vi "test_interpol.vi"() -> ()   [LabVIEW 2018]
uses:
  <vilib>/ptbypt/NI_PtbyPt.lvlib
panel:
  in  "sample length":i32=100
  in  "milliseconds to wait":u32
  in  "stop":bool
  out "Waveform Chart":dbl(graph)
  in  "x value":dbl format="%0.2f"
  in  "y":dbl format="%0.2f"
  out "Waveform Graph":dbl[](graph)
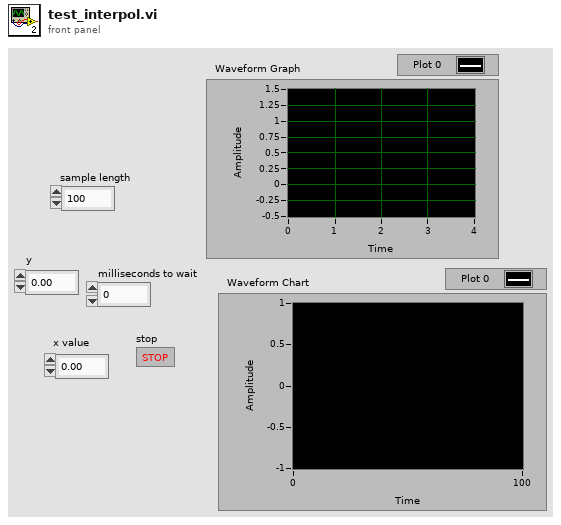
[diagram p1: front panel]
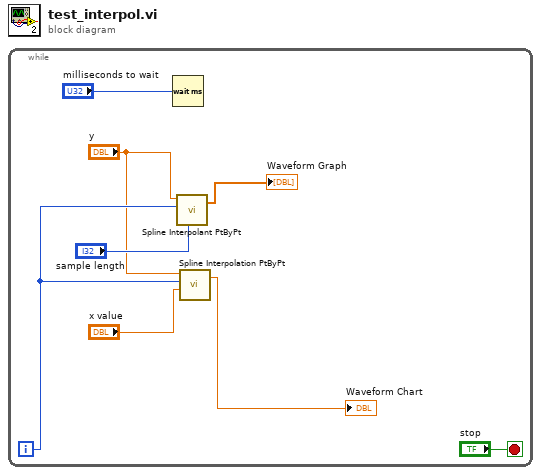
[diagram p0: block diagram]
diagram:
  n1 = while {
    i -> [w3]
    stop <- "stop" stop-if-true
    n2 = Wait (ms)(milliseconds to wait="milliseconds to wait") -> ()  [unwired: 1 out]
    n3 = call <vilib>:"Spline Interpolant PtByPt.vi"("sample length"="sample length", "x"=w3, "y"="y") -> ("Interpolant"=→"Waveform Graph":dbl[])  [unwired: 3 in, 1 out]
    n4 = call <vilib>:"Spline Interpolation PtByPt.vi"("x value"="x value", "x"=w3, "y"="y") -> ("interpolation value"=→"Waveform Chart":dbl)  [unwired: 3 in, 1 out]
  }
